vi "CSM-TCP-Router.vi"(7 "Name(\"\" to use uuid)":string="CSM TCP Router", 10 "Net Address(Empty for all Adaptor)":string, 11 "ServerInfo":T1={"Server.Port"=50007, "Server.MaxConnections"=10}) -> ()   [LabVIEW 2020, in "CSM-TCP-Router.lvlib"]
uses:
  CSM-TCP-Router.lvlib
  <vilib>/addons/_JKI.lib/_JKI_lib_TCP_Server.llb/JKI TCP Server.lvclass
  c1170cab-26a1-46e4-9ba3-f0b0422945de.vi
  216db8cf-36de-42cb-a8f5-94166053bff2.vi
  4e85c3fb-ef85-4e26-a42c-c5beb394b70a.vi
  3806dceb-3f37-4f57-9f18-971811feca89.vi
  205c1708-77cc-49ae-adf6-94a57fa2f451.vi
  585d93a8-ed6f-41ff-b581-bed18c521f0c.vi
  12c0d3a3-a730-47d2-a02c-5596bfd9aeb4.vi
  <userlib>/_NEVSTOP/Communicable State Machine(CSM)/AdvanceAPI/CSM - Revert Arguments-Safe String.vi
  <userlib>/_NEVSTOP/Communicable State Machine(CSM)/AdvanceAPI/CSM - Make String Arguments Safe.vi
  <userlib>/_NEVSTOP/Communicable State Machine(CSM)/AdvanceAPI/CSM - Break Down Multiple States String.vi
  <userlib>/_NEVSTOP/Communicable State Machine(CSM)/AdvanceAPI/CSM - Compact Multiple States.vi
  c1170cab-26a1-46e4-9ba3-f0b0422945de.vi/b09b9099-6be0-413b-8afc-4908471460c3.vi
  <userlib>/_NEVSTOP/Communicable State Machine(CSM)/addons/INI-Static-Variable-Support/_Support/FlagInstance-CSMINIVariable.vi
  216db8cf-36de-42cb-a8f5-94166053bff2.vi/b09b9099-6be0-413b-8afc-4908471460c3.vi
  <userlib>/_NEVSTOP/Communicable State Machine(CSM)/AdvanceAPI/CSM - Keywords.vi
  <userlib>/_NEVSTOP/Communicable State Machine(CSM)/_Support/ChangeFlag/ChangeFlag-Read.vi
  <userlib>/_NEVSTOP/Communicable State Machine(CSM)/_Shared/Trim Single-line Text.vi
  <userlib>/_NEVSTOP/Communicable State Machine(CSM)/_Support/ChangeFlag/ChangeFlagDB.vi
  <vilib>/Utility/Data Type/Get Type Information.vi
  <userlib>/_NEVSTOP/Communicable State Machine(CSM)/addons/API-String-Arugments-Support/_Support/Data To SingleElementsArray_csm.vi
  <userlib>/_NEVSTOP/Communicable State Machine(CSM)/addons/INI-Static-Variable-Support/_Support/Parse Used Session and Name.vi
  <userlib>/_NEVSTOP/Communicable State Machine(CSM)/addons/API-String-Arugments-Support/_Support/Data To API String Arguments.vi
  <userlib>/_NEVSTOP/Communicable State Machine(CSM)/addons/INI-Static-Variable-Support/_Support/INI-FGV(lvlibp).vi
  <userlib>/_NEVSTOP/Communicable State Machine(CSM)/addons/INI-Static-Variable-Support/_Support/Populate String with INI Variable.vi
  <userlib>/_NEVSTOP/Communicable State Machine(CSM)/addons/API-String-Arugments-Support/_Support/Convert API String Arguments to Data(variant).vi
  <userlib>/_NEVSTOP/Communicable State Machine(CSM)/addons/API-String-Arugments-Support/_Support/SingleElementsArray To Data_csm.vi
  <userlib>/_NEVSTOP/Communicable State Machine(CSM)/addons/API-String-Arugments-Support/_Support/Query Data as API String Arguments(variant).vi
  _support/Connection Handler Worker.vi
  <userlib>/_NEVSTOP/Communicable State Machine(CSM)/Communicable State Machine.lvlib
panel:
  out "Error Occurred":errorcluster
  out "State History":string
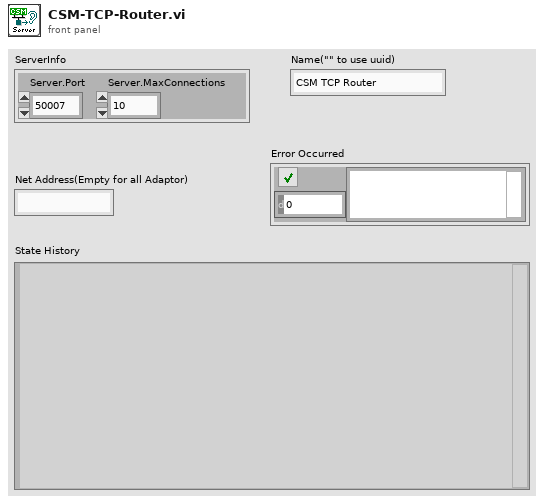
[diagram p1: front panel]
types:
  T1 = cluster{"Server.Port":u16, "Server.MaxConnections":u32}
  T2 = enum32{"Invalid", "Standard", "Closed", "Hidden", "Minimized", "Maximized"}
  T3 = enum32{"invalid app kind", "Development System", "Run Time System", "Student Edition", "Embedded LabVIEW", "Evaluation", "Custom"}
  T4 = typedef "Communicable State Machine.lvlib/_CSM_Response Source Message.ctl" = cluster{"‘State":string, "’Arguments":string, "’Error":errorcluster}
  T5 = cluster{"Current VI Reference":refnum<vi>, "Close Panel on Exit?":bool}
  T6 = cluster{"Core":cluster{"Current VI Reference":refnum<vi>, "Close Panel on Exit?":bool}, "ServerInfo":cluster{"Server.Port":u16, "Server.MaxConnections":u32}, "Address":string}
  T7 = typedef "JKI TCP Server.lvclass/TCP Server Public Connections Info Cluster.ctl" = cluster{"Remote Address":string, "remote port":u16, "time connected (s)":dbl}
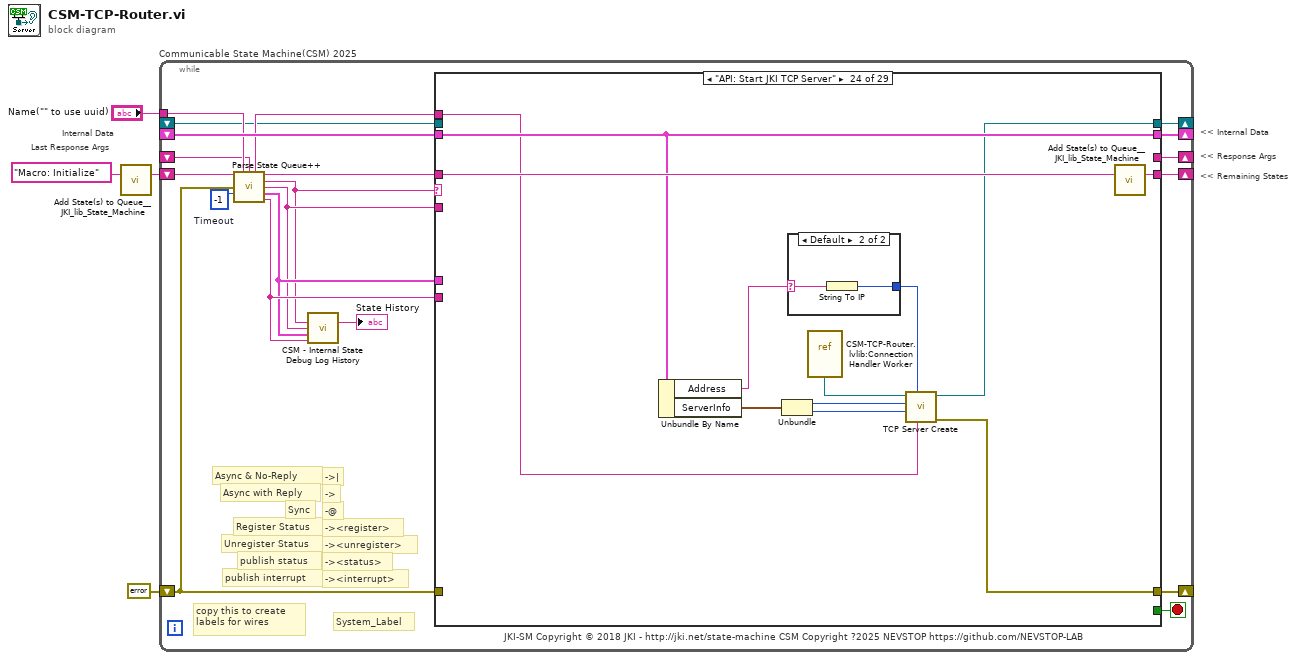
[diagram p0: block diagram]
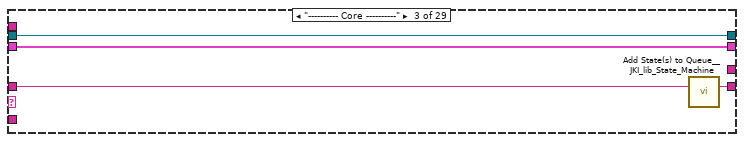
[diagram p4: hidden frame]
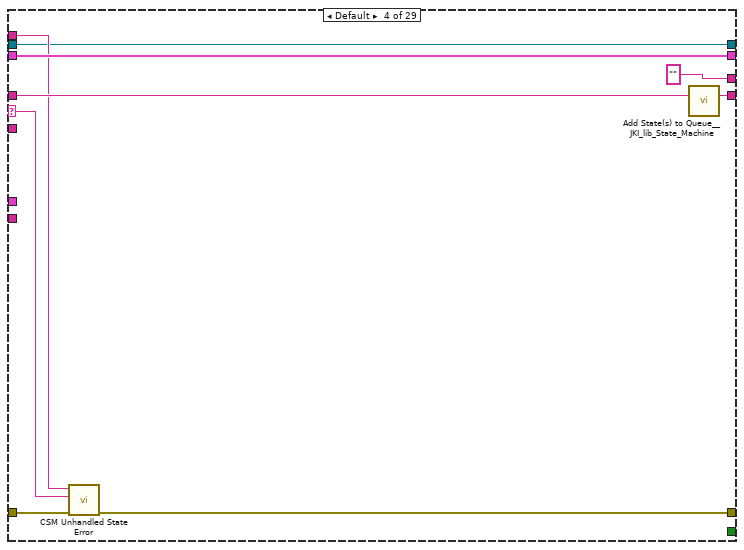
[diagram p5: hidden frame]
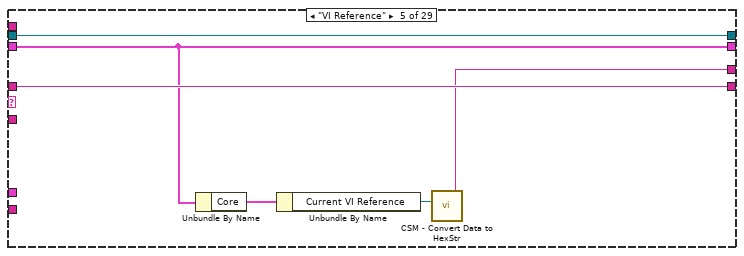
[diagram p6: hidden frame]
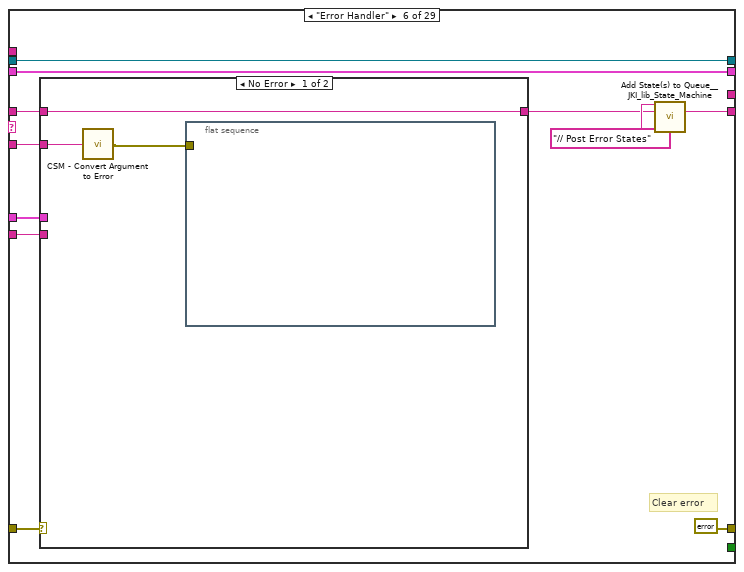
[diagram p7: hidden frame]
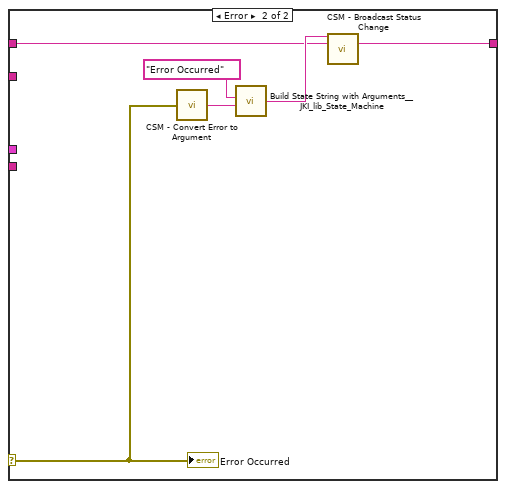
[diagram p8: hidden frame]
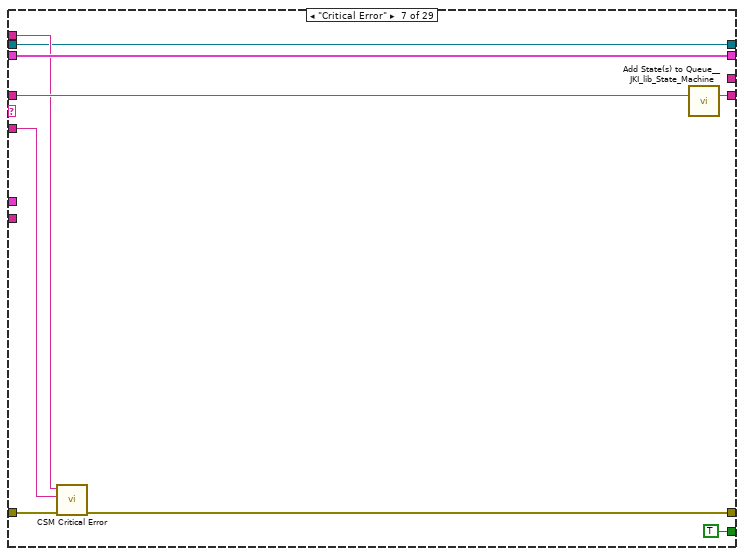
[diagram p9: hidden frame]
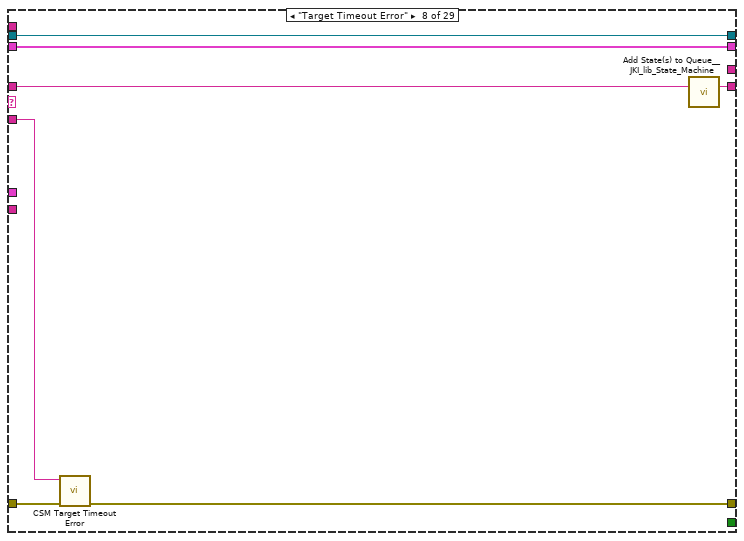
[diagram p10: hidden frame]
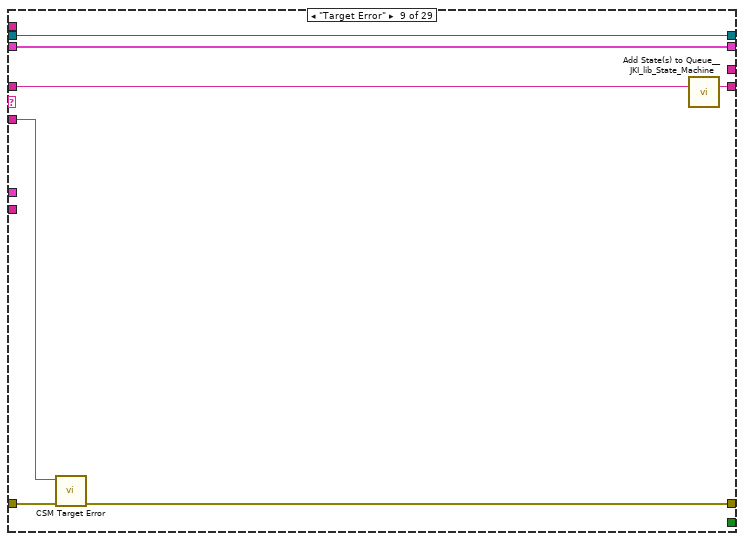
[diagram p11: hidden frame]
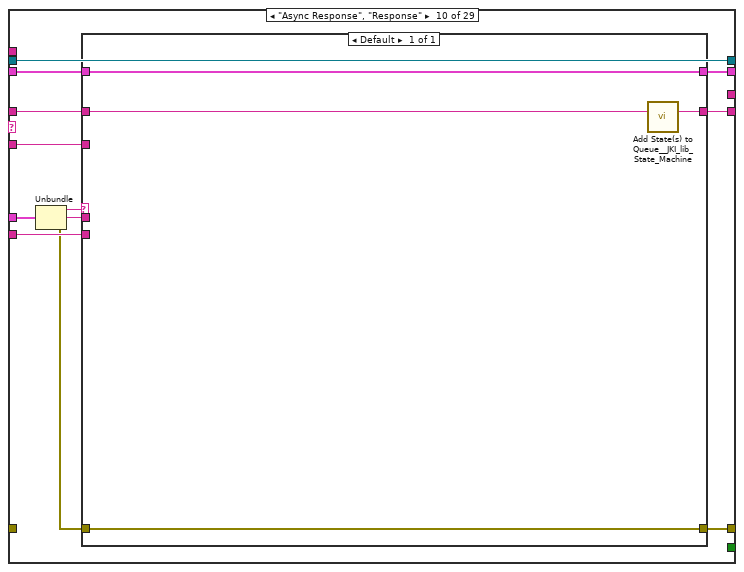
[diagram p12: hidden frame]
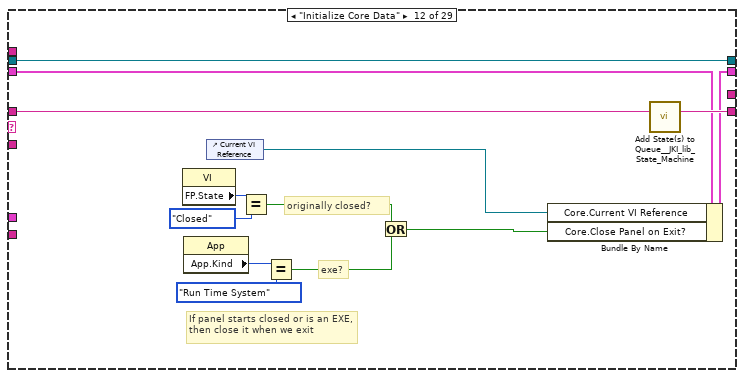
[diagram p14: hidden frame]
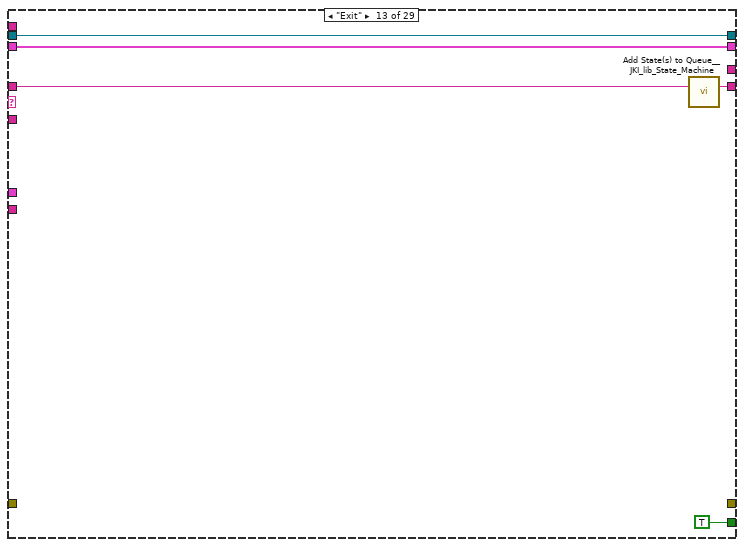
[diagram p15: hidden frame]
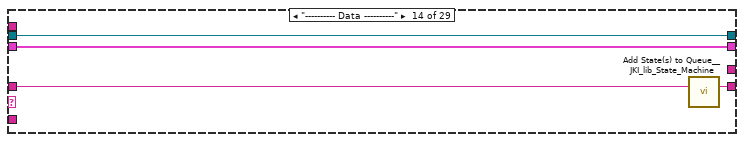
[diagram p16: hidden frame]
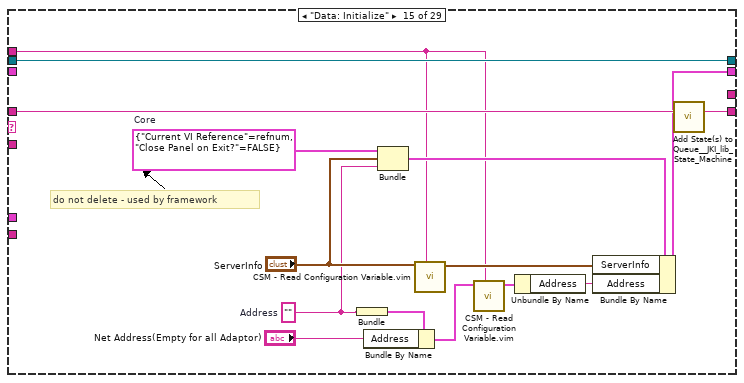
[diagram p17: hidden frame]
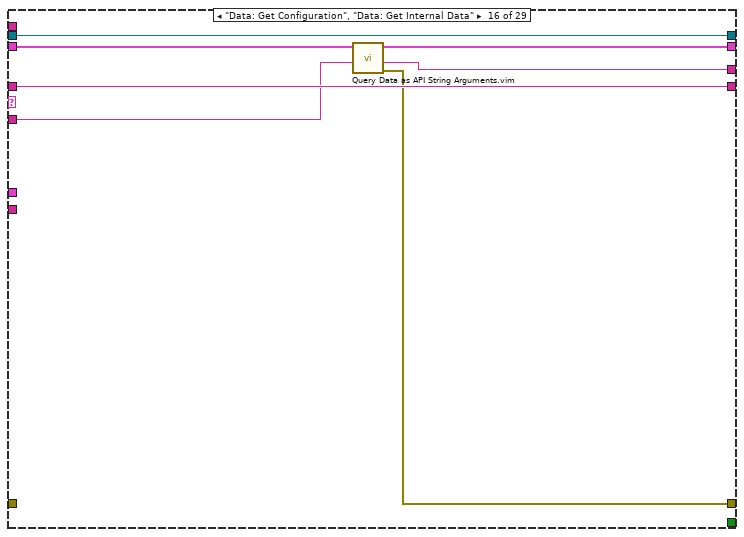
[diagram p18: hidden frame]
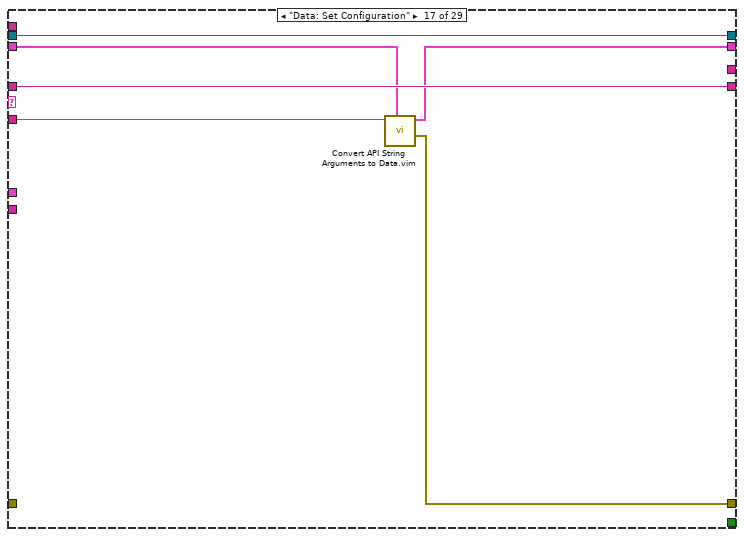
[diagram p19: hidden frame]
diagram:
  # "Last Response Args"
  # "Internal Data"
  # "<< Internal Data"
  # "<< Response Args"
  # "<< Remaining States"
  n1 = call <vilib>:"Add State(s) to Queue__JKI_lib_State_Machine.vi"("State(s) in (\"\")"="Macro: Initialize" ("Init States(\"Macro: Initialize\")")) -> ("States Out"=w2:string)  [unwired: 14 in]
  n2 = while "Communicable State Machine(CSM) 2025" {
    shift-right: [w19] -> _
    shift-left: _ -> [w18]
    shift-right: [w22] -> _
    shift-left: errorcluster {"status"=FALSE, "code"=0, "source"=""} ("error out") -> [w8]
    shift-right: [w21] -> _
    shift-left: w2 -> [w23]
    tunnel: "Name(\"\" to use uuid)" -> [w15]
    shift-right: [w16] -> _
    shift-left: _ -> [w10]
    shift-right: [w6] -> _
    shift-left: _ -> [w5]
    stop <- w20 stop-if-true
    w17 = -1  # Timeout
    # "copy this to create labels for wires"
    # "System_Label"
    # "-><interrupt>"
    # "-><status>"
    # "-><unregister>"
    # "-><register>"
    # "-@"
    # "->"
    # "->|"
    # "publish interrupt"
    # "publish status"
    # "Unregister Status"
    # "Register Status"
    # "Sync"
    # "Async with Reply"
    # "Async & No-Reply"
    # "JKI-SM Copyright © 2018 JKI - http://jki.net/state-machine CSM Copyright ?2025 NEVSTOP https://github.com/NEVSTOP-LAB"
    n3 = call <userlib>:"Parse State Queue++.vi"("State Queue"=w23, "Name (\"\" to Use UUID)"=w15, "Response Arguments"=w10, "Previous Error"=w8, "Dequeue (1 ms)"=w17) -> ("Name Used"=w9:string, "Remaining States"=w24:string, "Current State"=w11:string, "Arguments"=w12:string, "Additional Information"=w13:T4, "Source CSM"=w14:string)  [unwired: 5 in]
    n4 = call <userlib>:"CSM - Internal State Debug Log History.vi"("State"=w11, "Arguments (\"\")"=w12, ">> Response Source Message >>"=w13, "Source (\"\")"=w14) -> ("Debug Log"=→"State History":string)  [unwired: 11 in]
    n5 = case shown="\"API: Start JKI TCP Server\"" w11 {
      selector: w11 -> [_ _ _ w38 _ _ _ _ _ _ _ _ _ _ _ _ _ _ _ _ _ _ _ _ _ _ _ _ _]
      tunnel: w24 -> [w26 w30 w34 w41 w49 w54 w77 w84 w91 w98 w111 w124 w129 w133 w148 w155 w161 w164 w170 w174 w179 w184 w187 w199 w207 w215 w223 w231 w237]
      tunnel: w12 -> [_ _ _ _ _ w53 w71 w81 w88 w97 _ _ _ _ _ w150 w160 _ _ _ _ _ _ _ _ _ _ _ _]
      tunnel: w18 -> [w27 w29 w32 w39 w46 w59 w75 w82 w89 w99 w110 w118 w127 w131 _ w154 w159 w163 w166 w172 w177 w182 w186 w194 w206 w214 w222 w230 w235]
      tunnel: [_ _ _ w43 _ errorcluster {"status"=FALSE, "code"=0, "source"=""} ("error out") w78 w80 w87 w102 _ _ _ _ _ w151 w157 _ w167 _ _ _ _ w192 w202 w210 w218 w226 w232] -> w22
      tunnel: w8 -> [_ _ _ w42 _ w57 w73 w85 w92 _ _ _ _ _ _ _ _ _ _ _ _ _ _ _ _ _ _ _ _]
      tunnel: [w26 w30 w33 w40 w49 w55 w76 w83 w90 w100 w111 w123 w128 w132 w147 w155 w161 w164 w169 w173 w178 w183 w187 w198 w207 w215 w223 w231 w236] -> w21
      tunnel: [_ _ _ _ _ _ TRUE _ _ _ _ _ TRUE _ _ _ _ _ _ _ _ _ _ _ _ _ _ _ _] -> w20
      tunnel: [w27 w29 w32 w39 w46 w59 w75 w82 w89 w101 w110 w122 w127 w131 w142 w153 w158 w163 w166 w172 w177 w182 w186 w194 w206 w214 w222 w230 w235] -> w19
      tunnel: w14 -> [_ _ _ _ _ w52 _ _ _ w95 _ _ _ _ _ _ _ _ _ _ _ _ _ _ _ _ _ _ _]
      tunnel: w13 -> [_ _ _ _ _ w51 _ _ _ w96 _ _ _ _ _ _ _ _ _ _ _ _ _ _ _ _ _ _ _]
      tunnel: [_ _ _ "" w45 _ _ _ _ _ _ _ _ _ _ w152 _ _ _ _ _ _ _ _ "API1 Response" w209 w217 w225 _] -> w16
      tunnel: w9 -> [_ _ _ w36 _ _ w72 _ _ _ _ _ _ _ w136 _ _ _ _ _ _ _ _ w190 _ _ _ _ _]
      tunnel: [w25 w28 w31 w35 w44 w50 w70 w79 w86 w93 w109 w112 w125 w130 w144 w149 w156 w162 w165 w171 w175 w180 w185 w191 w203 w212 w220 w228 refnum<class "JKI TCP Server.lvclass"> refnum ("TCP Server")] -> w6
      tunnel: w5 -> [w25 w28 w31 w35 w44 w50 w70 w79 w86 w93 w109 w112 w125 w130 w144 w149 w156 w162 w165 w171 w175 w180 w185 _ w204 w213 w221 w229 w234]
      frame "", "Idle" {
      }
      frame "CSM Documentation" {
      }
      frame "---------- Core ----------" {
        n6 = call <vilib>:"Add State(s) to Queue__JKI_lib_State_Machine.vi"("State(s) in (\"\")"=w34) -> ("States Out"=w33:string)  [unwired: 14 in]
      }
      frame Default {
        n7 = call <userlib>:"CSM Unhandled State Error.vi"("error in (no error)"=w42, "Undefined State"=w38, "CSM Name"=w36) -> ("error out"=w43:errorcluster)  [unwired: 8 in]
        n8 = call <vilib>:"Add State(s) to Queue__JKI_lib_State_Machine.vi"("State(s) in (\"\")"=w41) -> ("States Out"=w40:string)  [unwired: 14 in]
      }
      frame "VI Reference" {
        n9 = Unbundle By Name(w46) -> ("Core"=w48:T5)
        n10 = Unbundle By Name(w48) -> ("Current VI Reference"=w47:refnum<vi>)
        n11 = call <userlib>:"CSM - Convert Data to HexStr.vi"("Variant"=w47) -> ("HEX String (0-9,A-F)"=w45:string)  [unwired: 8 in]
      }
      frame "Error Handler" {
        # "Clear error"
        n12 = case shown="No Error" w57 {
          selector: w57 -> [_ w64]
          tunnel: [w63 w66] -> w56
          tunnel: w54 -> [w63 w65]
          tunnel: w53 -> [w62 _]
          tunnel: w52 -> [_ _]
          tunnel: w51 -> [_ _]
          frame No Error {
            n13 = call <userlib>:"CSM - Convert Argument to Error.vi"("Argument"=w62) -> ("Error"=w61:errorcluster)  [unwired: 4 in]
            n14 = flat-sequence {
              tunnel: w61 -> [_]
              frame #0 {
              }
            }
          }
          frame Error {
            n15 = call <userlib>:"CSM - Convert Error to Argument.vi"("Error"=w64) -> ("Argument"=w68:string)  [unwired: 4 in]
            n16 = call <vilib>:"Build State String with Arguments__JKI_lib_State_Machine.vi"("Arguments (\"\")"=w68, "State"="Error Occurred" ("Status with Arguments")) -> ("State with Arguments"=w67:string)  [unwired: 4 in]
            n17 = call <userlib>:"CSM - Broadcast Status Change.vi"("Status With Arguments"=w67, "State Queue"=w65) -> ("Remaining States"=w66:string)  [unwired: 13 in]
            "Error Occurred" <- w64
          }
        }
        n18 = call <vilib>:"Add State(s) to Queue__JKI_lib_State_Machine.vi"("State(s) in Front (\"\")"="// Post Error States", "State(s) in (\"\")"=w56) -> ("States Out"=w55:string)  [unwired: 13 in]
      }
      frame "Critical Error" {
        n19 = call <userlib>:"CSM Critical Error.vi"("error in (no error)"=w73, "Arugments (As Reason)"=w71, "CSM Name"=w72) -> ("error out"=w78:errorcluster)  [unwired: 8 in]
        n20 = call <vilib>:"Add State(s) to Queue__JKI_lib_State_Machine.vi"("State(s) in (\"\")"=w77) -> ("States Out"=w76:string)  [unwired: 14 in]
      }
      frame "Target Timeout Error" {
        n21 = call <userlib>:"CSM Target Timeout Error.vi"("error in (no error)"=w85, "Arguments (As CSM Name)"=w81) -> ("error out"=w80:errorcluster)  [unwired: 9 in]
        n22 = call <vilib>:"Add State(s) to Queue__JKI_lib_State_Machine.vi"("State(s) in (\"\")"=w84) -> ("States Out"=w83:string)  [unwired: 14 in]
      }
      frame "Target Error" {
        n23 = call <userlib>:"CSM Target Error.vi"("error in (no error)"=w92, "Arguments (As CSM Name)"=w88) -> ("error out"=w87:errorcluster)  [unwired: 9 in]
        n24 = call <vilib>:"Add State(s) to Queue__JKI_lib_State_Machine.vi"("State(s) in (\"\")"=w91) -> ("States Out"=w90:string)  [unwired: 14 in]
      }
      frame "Async Response", "Response" {
        n25 = Unbundle(w96) -> ("‘State"=w104:string, "’Arguments"=w103:string, "’Error"=w94:errorcluster)
        n26 = case shown="Default" w104 {
          tunnel: [w105] -> w100
          tunnel: w98 -> [w106]
          tunnel: [w108] -> w101
          tunnel: w99 -> [w108]
          tunnel: [w107] -> w102
          tunnel: w94 -> [w107]
          tunnel: w95 -> [_]
          tunnel: w97 -> [_]
          tunnel: w103 -> [_]
          frame Default {
            n27 = call <vilib>:"Add State(s) to Queue__JKI_lib_State_Machine.vi"("State(s) in (\"\")"=w106) -> ("States Out"=w105:string)  [unwired: 14 in]
          }
        }
      }
      frame "Async Message Posted" {
      }
      frame "Initialize Core Data" {
        # "originally closed?"
        # "exe?"
        # "If panel starts closed or is an EXE, then close it when we exit"
        n28 = property class="VI"() -> ("FP.State"=w115:T2)  [unwired: 2 in, 2 out]
        n29 = property class="App"() -> ("App.Kind"=w121:T3)  [unwired: 2 in, 2 out]
        n30 = control-ref of="Current VI Reference"() -> (w116:refnum<vi>)
        n31 = Equal?(x=w115, y=T2."Closed" ("Front Panel Window:State")) -> (x = y?=w113:bool)
        n32 = Equal?(x=w121, y=T3."Run Time System" ("Application:Kind")) -> (x = y?=w119:bool)
        n33 = Or(x=w113, y=w119) -> (x .or. y?=w117:bool)
        n34 = Bundle By Name(cluster=w118, "Core.Current VI Reference"=w116, "Core.Close Panel on Exit?"=w117) -> (w122:T6)
        n35 = call <vilib>:"Add State(s) to Queue__JKI_lib_State_Machine.vi"("State(s) in (\"\")"=w124) -> ("States Out"=w123:string)  [unwired: 14 in]
      }
      frame "Exit" {
        n36 = call <vilib>:"Add State(s) to Queue__JKI_lib_State_Machine.vi"("State(s) in (\"\")"=w129) -> ("States Out"=w128:string)  [unwired: 14 in]
      }
      frame "---------- Data ----------" {
        n37 = call <vilib>:"Add State(s) to Queue__JKI_lib_State_Machine.vi"("State(s) in (\"\")"=w133) -> ("States Out"=w132:string)  [unwired: 14 in]
      }
      frame "Data: Initialize" {
        w140 = ""  # Address
        w145 = T5 {"Current VI Reference"=refnum, "Close Panel on Exit?"=FALSE}  # Core
        # "do not delete - used by framework"
        n38 = Bundle("Address"=w140) -> (w139:cluster{"Address":string})  [unwired: 1 in]
        n39 = Bundle By Name(cluster=w139, "Address"="Net Address(Empty for all Adaptor)") -> (w137:cluster{"Address":string})
        n40 = Bundle("Core"=w145, "ServerInfo"="ServerInfo", "Address"=w140) -> (w146:T6)  [unwired: 1 in]
        n41 = call "CSM - Read Configuration Variable.vim"("Section Name (\"\" as Default)"=w136, "Configuration Prototype (Cluster Prefered)"="ServerInfo") -> ("Configuration"=w141:T1)  [unwired: 6 in, 1 out]
        n42 = call "CSM - Read Configuration Variable.vim"("Section Name (\"\" as Default)"=w136, "Configuration Prototype (Cluster Prefered)"=w137) -> ("Configuration"=w135:cluster{"Address":string})  [unwired: 6 in, 1 out]
        n43 = Unbundle By Name(w135) -> ("Address"=w134:string)
        n44 = Bundle By Name(cluster=w146, "ServerInfo"=w141, "Address"=w134) -> (w142:T6)
        n45 = call <vilib>:"Add State(s) to Queue__JKI_lib_State_Machine.vi"("State(s) in (\"\")"=w148) -> ("States Out"=w147:string)  [unwired: 14 in]
      }
      frame "Data: Get Configuration", "Data: Get Internal Data" {
        n46 = call "Query Data as API String Arguments.vim"("Name"=w150, "Cluster Data"=w154) -> ("error"=w151:errorcluster, "API String"=w152:string, "Cluster Data (dup)"=w153:T6)  [unwired: 7 in]
      }
      frame "Data: Set Configuration" {
        n47 = call "Convert API String Arguments to Data.vim"("Reference Type"=w159, "API String"=w160) -> ("error out"=w157:errorcluster, "Data"=w158:T6)  [unwired: 6 in]
      }
      frame "Data: Update Indicators" {
      }
      frame "Data: Cleanup" {
        n48 = Unbundle By Name(w166) -> ("Core.Current VI Reference"=w168:refnum<vi>)
        n49 = Close Reference(reference=w168) -> (error out=w167:errorcluster)  [unwired: 1 in]
        n50 = call <vilib>:"Add State(s) to Queue__JKI_lib_State_Machine.vi"("State(s) in (\"\")"=w170) -> ("States Out"=w169:string)  [unwired: 14 in]
      }
      frame "---------- Macro ----------" {
        n51 = call <vilib>:"Add State(s) to Queue__JKI_lib_State_Machine.vi"("State(s) in (\"\")"=w174) -> ("States Out"=w173:string)  [unwired: 14 in]
      }
      frame "Macro: Initialize" {
        n52 = call <vilib>:"Add State(s) to Queue__JKI_lib_State_Machine.vi"("State(s) in Front (\"\")"="Data: Initialize\nInitialize Core Data\nData: Update Indicators\nAPI: Start JKI TCP Server", "State(s) in (\"\")"=w179) -> ("States Out"=w178:string)  [unwired: 13 in]
      }
      frame "Macro: Exit" {
        n53 = call <vilib>:"Add State(s) to Queue__JKI_lib_State_Machine.vi"("State(s) in Front (\"\")"="API: Stop JKI TCP Server\nData: Cleanup\nExit", "State(s) in (\"\")"=w184) -> ("States Out"=w183:string)  [unwired: 13 in]
      }
      frame "---------- API ----------" {
      }
      frame "API: Start JKI TCP Server" {
        n54 = Unbundle By Name(w194) -> ("Address"=w188:string, "ServerInfo"=w193:T1)
        n55 = Unbundle(w193) -> ("Server.Port"=w195:u16, "Server.MaxConnections"=w197:u32)
        n56 = case shown="Default" w188 {
          selector: w188 -> [_ w200]
          tunnel: [_ w201] -> w189
          frame "" {
          }
          frame Default {
            n57 = String To IP(1:w200) -> (0:w201:u32)
          }
        }
        n58 = vi-ref "CSM-TCP-Router.lvlib:Connection Handler Worker.vi"() -> ("vi reference"=w196:refnum<vi>)
        n59 = call <vilib>:"TCP Server Create.vi"("Additional Data"=w190, "net address (0: Listen on All Adaptors)"=w189, "max connections (0: no limit)"=w197, "port"=w195, "Connection Handler Call-Back VI RefNum"=w196) -> ("error out"=w192:errorcluster, "TCP Server"=w191:refnum<class "JKI TCP Server.lvclass">)  [unwired: 5 in]
        n60 = call <vilib>:"Add State(s) to Queue__JKI_lib_State_Machine.vi"("State(s) in (\"\")"=w199) -> ("States Out"=w198:string)  [unwired: 14 in]
      }
      frame "API: Disconnect All Client" {
        n61 = call <vilib>:"TCP Disconnect All Clients.vi"("TCP Server"=w204) -> ("error out"=w202:errorcluster, "TCP Server out"=w203:refnum<class "JKI TCP Server.lvclass">)  [unwired: 9 in]
      }
      frame "API: Get Time Running" {
        n62 = call <vilib>:"TCP Server Get Connections Info.vi"("TCP Server"=w213) -> ("error out"=w211:errorcluster, "TCP Server out"=w212:refnum<class "JKI TCP Server.lvclass">, "time running (s)"=w208:dbl)  [unwired: 6 in, 2 out]
        n63 = call "Convert Data To API String Arguments.vim"("error in (no error)"=w211, "Data"=w208) -> ("error out"=w210:errorcluster, "API String"=w209:string)  [unwired: 6 in]
      }
      frame "API: Get Connection Number" {
        n64 = call <vilib>:"TCP Server Get Connections Info.vi"("TCP Server"=w221) -> ("error out"=w219:errorcluster, "Number of Connections"=w216:u32, "TCP Server out"=w220:refnum<class "JKI TCP Server.lvclass">)  [unwired: 6 in, 2 out]
        n65 = call "Convert Data To API String Arguments.vim"("error in (no error)"=w219, "Data"=w216) -> ("error out"=w218:errorcluster, "API String"=w217:string)  [unwired: 6 in]
      }
      frame "API: Get Connection Details" {
        n66 = call <vilib>:"TCP Server Get Connections Info.vi"("TCP Server"=w229) -> ("error out"=w227:errorcluster, "Connections Info"=w224:T7[], "TCP Server out"=w228:refnum<class "JKI TCP Server.lvclass">)  [unwired: 6 in, 2 out]
        n67 = call "Convert Data To API String Arguments.vim"("error in (no error)"=w227, "Data"=w224) -> ("error out"=w226:errorcluster, "API String"=w225:string)  [unwired: 6 in]
      }
      frame "API: Stop JKI TCP Server" {
        n68 = call <vilib>:"TCP Server Destroy.vi"("TCP Server"=w234) -> ("error out"=w232:errorcluster)  [unwired: 10 in]
        n69 = call <vilib>:"Add State(s) to Queue__JKI_lib_State_Machine.vi"("State(s) in (\"\")"=w237) -> ("States Out"=w236:string)  [unwired: 14 in]
      }
    }
  }
